vi "Intake Balls.vi"(10 "Enum":enum16{"Do Nothing", "Down", "Up"}(ring)) -> ()   [LabVIEW 2018]
uses:
  <vilib>/Rock Robotics/WPI/ThirdParty/Phoenix-LabVIEW/Motor Controller/Controls/CTRE_Phoenix_MotorControl_ControlMode.ctl
  Refnums.vi
  <vilib>/Rock Robotics/WPI/ThirdParty/Phoenix-LabVIEW/Motor Controller/Get/CTRE_Phoenix_MotorController_GetQuadratureData.vi
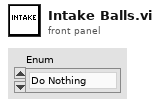
[diagram p1: front panel]
types:
  T1 = typedef "WPI_RobotDriveDevRef.ctl" = cluster{"DevStatus":errorcluster, "Motors[]":T2[], "Square Inputs":bool, "Max Output":dbl}
  T2 = typedef "WPI_MotorControlDeviceRef.ctl" = cluster{"DeviceStatus":errorcluster, "Type":T3, "PWM":cluster{"PWM Channel":T4, "DeadBand":T5}, "CAN":cluster{"Device Number":u8, "SetOutput VI Ref":variant, "GetOutput VI Ref":variant, "Enable VI Ref":variant, "Disable VI Ref":variant, "Data":variant}, "Invert":bool, "DIO PWM":cluster{"PWM \"Enable\" Channel":T4, "DIOChannel":T6, "PWM Rate":dbl}}
  T3 = typedef "WPI_MotorControlType.ctl" = enum16{"PWM", "CAN", "DIO PWM"}
  T4 = typedef "FPGA_DIOPWMChannel.ctl" = enum8{"PWM 0", "PWM 1", "PWM 2", "PWM 3", "PWM 4", "PWM 5", "PWM 6", "PWM 7", "PWM 8", "PWM 9", "PWM MXP 0", "PWM MXP 1", "PWM MXP 2", "PWM MXP 3", "PWM MXP 4", "PWM MXP 5", "PWM MXP 6", "PWM MXP 7", "PWM MXP 8", "PWM MXP 9", "Invalid"}
  T5 = typedef "WPI_PWMDeadband.ctl" = cluster{"Name":string, "maxPositivePwm":i32, "minPositivePwm":i32, "centerPwm":i32, "maxNegativePwm":i32, "minNegativePwm":i32, "angularRange":u16}
  T6 = typedef "FPGA_DIOChannel.ctl" = enum8{"DIO 0", "DIO 1", "DIO 2", "DIO 3", "DIO 4", "DIO 5", "DIO 6", "DIO 7", "DIO 8", "DIO 9", "DIO MXP 0", "DIO MXP 1", "DIO MXP 2", "DIO MXP 3", "DIO MXP 4", "DIO MXP 5", "DIO MXP 6", "DIO MXP 7", "DIO MXP 8", "DIO MXP 9", "DIO MXP 10", "DIO MXP 11", "DIO MXP 12", "DIO MXP 13", "DIO MXP 14", "DIO MXP 15", "SPI Port CS1", "SPI Port CS2", "SPI Port CS3", "SPI Port MISO", "SPI Port MOSI", "Invalid"}
  T7 = cluster{"DriveTrain":T1, "LeftDrive":T2, "RightDrive":T2, "Elevator":T2, "Pivot":T2, "Intake":T2, "Right Climber":T2, "Left Climber":T2, "Shooter":T2}
  T8 = typedef "CTRE_Phoenix_MotorControl_ControlMode.ctl" = u16
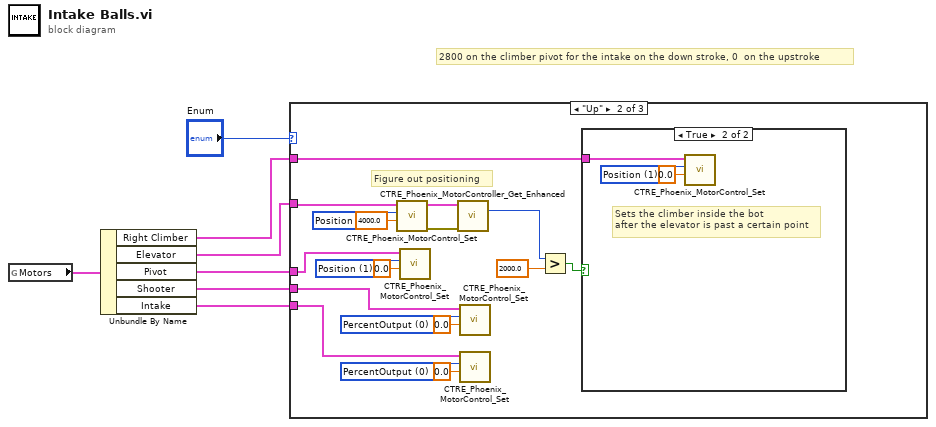
[diagram p0: block diagram]
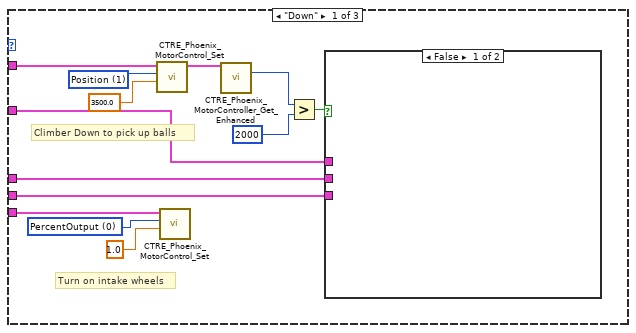
[diagram p2: hidden frame]
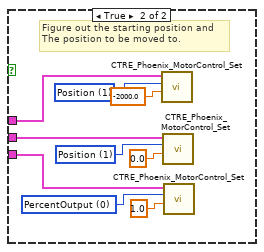
[diagram p3: hidden frame]
diagram:
  # "2800 on the climber pivot for the intake on the down stroke, 0  on the upstroke"
  n1 = global read "Refnums.vi" "Motors"() -> (w7:T7)
  n2 = Unbundle By Name(w7) -> ("Right Climber"=w6:T2, "Elevator"=w5:T2, "Pivot"=w4:T2, "Shooter"=w3:T2, "Intake"=w2:T2)
  n3 = case shown="\"Up\"" "Enum" {
    tunnel: w6 -> [w20 w38 _]
    tunnel: w5 -> [w13 w47 _]
    tunnel: w4 -> [w12 w42 _]
    tunnel: w3 -> [w11 w31 _]
    tunnel: w2 -> [w9 w30 _]
    frame "Down" {
      w8 = T8 0 items=["PercentOutput"=0, "Position"=1, "Velocity"=2, "Current"=3, "Follower"=5, "MotionProfile"=6, "MotionMagic"=7, "MotionProfileArc"=10, "Disabled"=15] ("Control Mode")
      w19 = T8 1 items=["PercentOutput"=0, "Position"=1, "Velocity"=2, "Current"=3, "Follower"=5, "MotionProfile"=6, "MotionMagic"=7, "MotionProfileArc"=10, "Disabled"=15] ("Control Mode")
      # "Turn on intake wheels"
      # "Climber Down to pick up balls"
      n4 = call <vilib>:"CTRE_Phoenix_MotorControl_Set.vi"("Output"=3500.0, "Control Mode"=w19, "PhoenixMotorControlDevRef"=w20) -> ("PhoenixMotorControlDevRef"=w17:T2)  [unwired: 7 in, 1 out]
      n5 = call <vilib>:"CTRE_Phoenix_MotorControl_Set.vi"("Output"=1.0, "Control Mode"=w8, "PhoenixMotorControlDevRef"=w9) -> ()  [unwired: 7 in, 2 out]
      n6 = call-poly <vilib>:"CTRE_Phoenix_MotorController_Get_Enhanced.vi"("PhoenixMotorControlDevRef"=w17) -> ("Quadrature Position"=w15:i32)  [unwired: 11 in, 3 out]
      n7 = Greater?(x=w15, y=2000) -> (0:w16:bool)
      n8 = case shown="False" w16 {
        tunnel: w13 -> [_ w28]
        tunnel: w12 -> [_ w25]
        tunnel: w11 -> [_ w21]
        frame False {
        }
        frame True {
          w22 = T8 0 items=["PercentOutput"=0, "Position"=1, "Velocity"=2, "Current"=3, "Follower"=5, "MotionProfile"=6, "MotionMagic"=7, "MotionProfileArc"=10, "Disabled"=15] ("Control Mode")
          w24 = T8 1 items=["PercentOutput"=0, "Position"=1, "Velocity"=2, "Current"=3, "Follower"=5, "MotionProfile"=6, "MotionMagic"=7, "MotionProfileArc"=10, "Disabled"=15] ("Control Mode")
          w29 = T8 1 items=["PercentOutput"=0, "Position"=1, "Velocity"=2, "Current"=3, "Follower"=5, "MotionProfile"=6, "MotionMagic"=7, "MotionProfileArc"=10, "Disabled"=15] ("Control Mode")
          # "Figure out the starting position and\nThe position to be moved to."
          n9 = call <vilib>:"CTRE_Phoenix_MotorControl_Set.vi"("Output"=-2000.0, "Control Mode"=w29, "PhoenixMotorControlDevRef"=w28) -> ()  [unwired: 7 in, 2 out]
          n10 = call <vilib>:"CTRE_Phoenix_MotorControl_Set.vi"("Output"=0.0, "Control Mode"=w24, "PhoenixMotorControlDevRef"=w25) -> ()  [unwired: 7 in, 2 out]
          n11 = call <vilib>:"CTRE_Phoenix_MotorControl_Set.vi"("Output"=1.0, "Control Mode"=w22, "PhoenixMotorControlDevRef"=w21) -> ()  [unwired: 7 in, 2 out]
        }
      }
    }
    frame "Up" {
      w33 = T8 0 items=["PercentOutput"=0, "Position"=1, "Velocity"=2, "Current"=3, "Follower"=5, "MotionProfile"=6, "MotionMagic"=7, "MotionProfileArc"=10, "Disabled"=15] ("Control Mode")
      w35 = T8 0 items=["PercentOutput"=0, "Position"=1, "Velocity"=2, "Current"=3, "Follower"=5, "MotionProfile"=6, "MotionMagic"=7, "MotionProfileArc"=10, "Disabled"=15] ("Control Mode")
      w37 = T8 1 items=["PercentOutput"=0, "Position"=1, "Velocity"=2, "Current"=3, "Follower"=5, "MotionProfile"=6, "MotionMagic"=7, "MotionProfileArc"=10, "Disabled"=15] ("Control Mode")
      w46 = T8 1 items=["PercentOutput"=0, "Position"=1, "Velocity"=2, "Current"=3, "Follower"=5, "MotionProfile"=6, "MotionMagic"=7, "MotionProfileArc"=10, "Disabled"=15] ("Control Mode")
      # "Figure out positioning"
      n12 = call <vilib>:"CTRE_Phoenix_MotorControl_Set.vi"("Output"=4000.0, "Control Mode"=w46, "PhoenixMotorControlDevRef"=w47) -> ("error out"=w43:errorcluster, "PhoenixMotorControlDevRef"=w44:T2)  [unwired: 7 in]
      n13 = call <vilib>:"CTRE_Phoenix_MotorControl_Set.vi"("Output"=0.0, "Control Mode"=w37, "PhoenixMotorControlDevRef"=w42) -> ()  [unwired: 7 in, 2 out]
      n14 = call-poly <vilib>:"CTRE_Phoenix_MotorController_Get_Enhanced.vi"("PhoenixMotorControlDevRef"=w44, "error in"=w43) -> ("Quadrature Position"=w39:i32)  [unwired: 10 in, 3 out]
      n15 = call <vilib>:"CTRE_Phoenix_MotorControl_Set.vi"("Output"=0.0, "Control Mode"=w33, "PhoenixMotorControlDevRef"=w31) -> ()  [unwired: 7 in, 2 out]
      n16 = call <vilib>:"CTRE_Phoenix_MotorControl_Set.vi"("Output"=0.0, "Control Mode"=w35, "PhoenixMotorControlDevRef"=w30) -> ()  [unwired: 7 in, 2 out]
      n17 = Greater?(x=w39, y=2000.0) -> (0:w41:bool)
      n18 = case shown="True" w41 {
        tunnel: w38 -> [_ w48]
        frame False {
        }
        frame True {
          w50 = T8 1 items=["PercentOutput"=0, "Position"=1, "Velocity"=2, "Current"=3, "Follower"=5, "MotionProfile"=6, "MotionMagic"=7, "MotionProfileArc"=10, "Disabled"=15] ("Control Mode")
          # "Sets the climber inside the bot\nafter the elevator is past a certain point"
          n19 = call <vilib>:"CTRE_Phoenix_MotorControl_Set.vi"("Output"=0.0, "Control Mode"=w50, "PhoenixMotorControlDevRef"=w48) -> ()  [unwired: 7 in, 2 out]
        }
      }
    }
    frame "Do Nothing", Default {
    }
  }
